vi "Actor Core.vi"(8 "error in":errorcluster, 11 "Chat Window in":refnum<class "Chat Window.lvclass">) -> (0 "error out":errorcluster, 3 "Actor out":refnum<class "Actor.lvclass">)   [LabVIEW 2020, in "Chat Window.lvlib" / "Chat Window.lvclass"]
doc: "(<B>Filename</B>: Actor Framework.lvlib:Actor.lvclass:Actor Core.vi)\n\nReceives messages to the actor, reacts to them, and initiates any error handling that may shut the actor down.\n\nDescendant classes may override this VI to append parallel tasks for the actor to complete while it handles messages. Overrides use the Call Parent Method node."
uses:
  Chat Window.lvclass
  C:/Program Files (x86)/National Instruments/LabVIEW 2020/vi.lib/ActorFramework/Actor/Actor.lvclass
  <vilib>/ActorFramework/Actor/Actor.lvclass
  <vilib>/NI/Actors/Network Endpoint Actors/Notifying Nested Endpoint/Notifying Nested Endpoint.lvclass
  G:/Utilisateurs/hugofroylan.aragon/Documents/Nested Endpoint Actors Optimized/Network Endpoint/Network Endpoint/Network Endpoint.lvclass
  Chat Window.lvclass/Chat Window.ctl
  Nested Endpoint Actors/Network Endpoint/Network Endpoint/Network Endpoint.lvclass/Network Endpoint.ctl
  <vilib>/ActorFramework/Actor/Actor.lvclass/Actor.ctl
  <vilib>/ActorFramework/Message Enqueuer/Message Enqueuer.lvclass/Message Enqueuer.ctl
  Chat Window Messages/Display Text Msg/Display Text Msg.lvclass/Display Text Msg.ctl
  Chat Window Messages/Update Number Msg/Update Number Msg.lvclass/Update Number Msg.ctl
  <vilib>/ActorFramework/Message Enqueuer/Init from Existing Queue.vi
  <vilib>/ActorFramework/Message Enqueuer/Enqueue.vi
  Chat Window Messages/Display Text Msg/Display Text Msg.lvclass
  C:/Program Files (x86)/National Instruments/LabVIEW 2020/vi.lib/ActorFramework/Message/Message.lvclass
  Chat Window Messages/Update Number Msg/Update Number Msg.lvclass
  <vilib>/ActorFramework/Stop Msg/Stop Msg.lvclass
  <vilib>/ActorFramework/Message Priority Queue/Priority Enqueue.vi
  <vilib>/ActorFramework/Message Enqueuer/Message Enqueuer.lvclass
  Nested Endpoint Actors/Network Endpoint/Network Endpoint/Network Endpoint.lvclass
panel:
  out "Text to display 2":string
  in  "Send echo":bool
  out "Number":dbl
  out "Connected":bool
  in  "Send":bool
  out "Text to display":string
  in  "Text to send":string
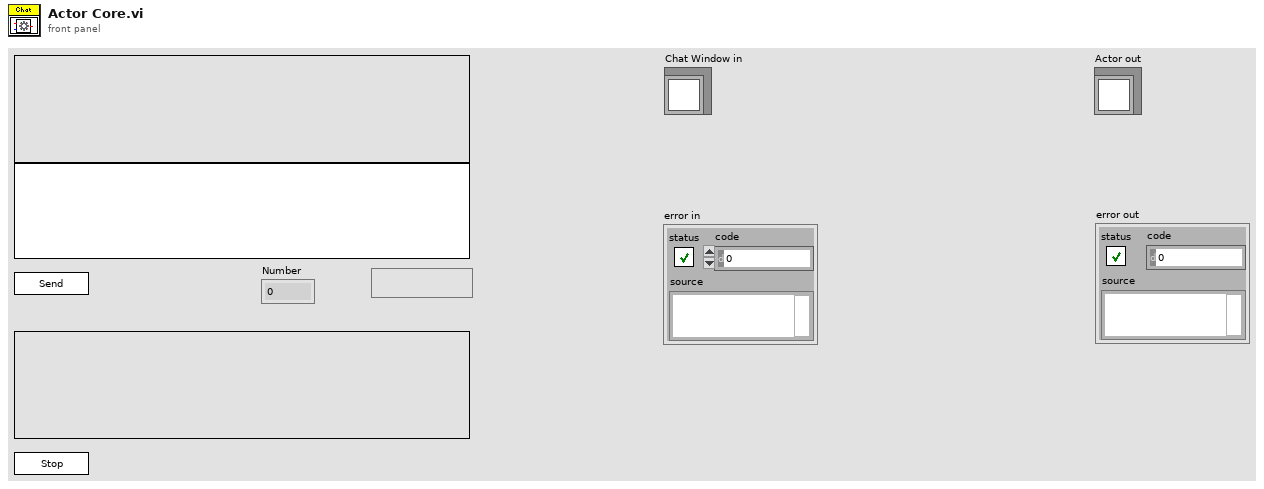
[diagram p1: front panel]
types:
  T1 = cluster{"Stop":refnum<user-event>, "Text":refnum<user-event>, "Connected":refnum<user-event>, "Number":refnum<user-event>, "echo":refnum<user-event>}
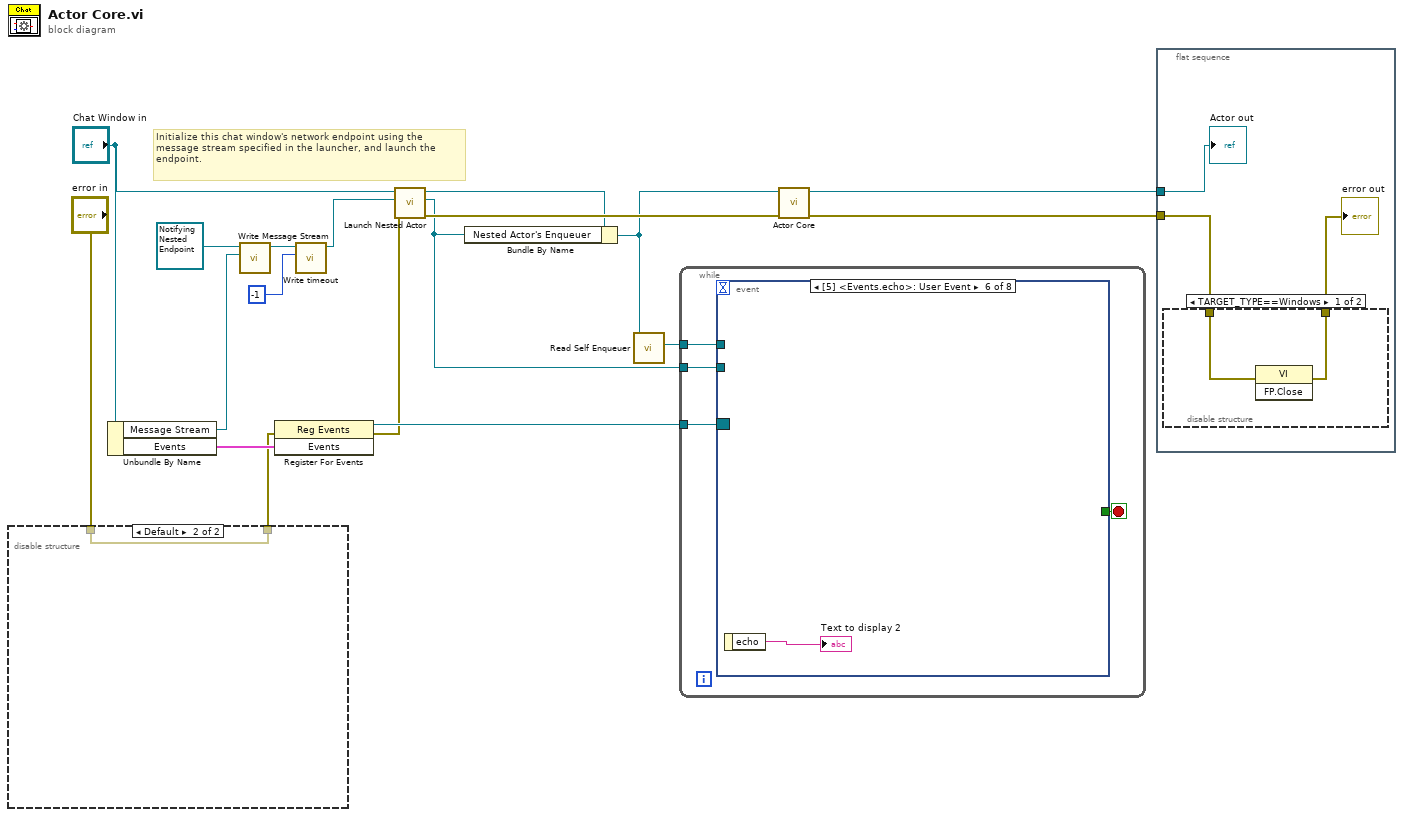
[diagram p0: block diagram]
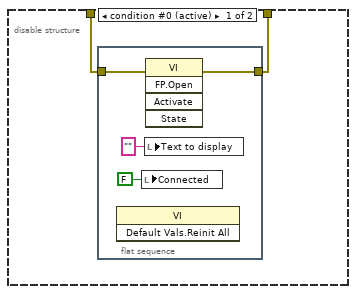
[diagram p2: hidden frame]
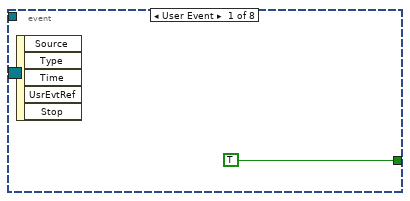
[diagram p4: hidden frame]
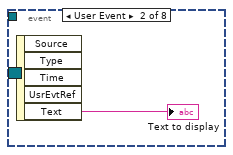
[diagram p5: hidden frame]
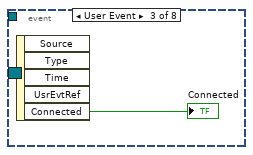
[diagram p6: hidden frame]
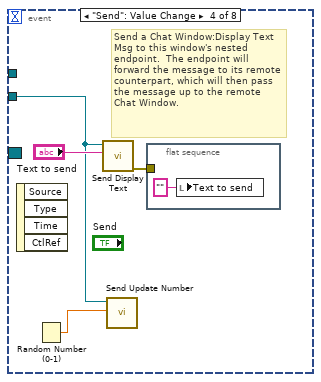
[diagram p7: hidden frame]
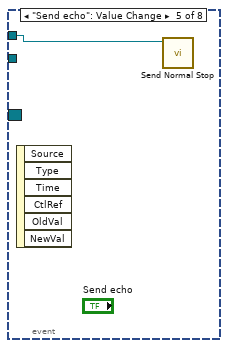
[diagram p8: hidden frame]
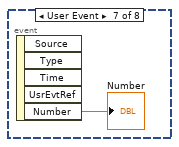
[diagram p9: hidden frame]
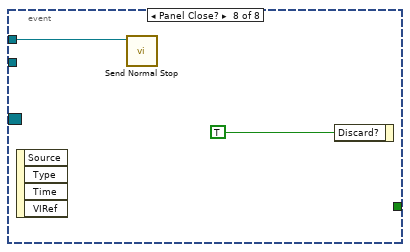
[diagram p10: hidden frame]
diagram:
  # "Initialize this chat window's network endpoint using the message stream specified in the launcher, and launch the endpoint."
  n1 = disable-structure shown="Default" {
    disable-tunnel: [w20 w25] -> w11
    disable-tunnel: "error in" -> [w19 w25]
    frame condition #0 (active) {
      n2 = flat-sequence {
        tunnel: [w24] -> w20
        tunnel: w19 -> [w21]
        frame #0 {
          n3 = invoke class="VI" method="Default Vals.Reinit All"() -> ()  [unwired: 3 in, 3 out]
          n4 = local write "Connected"(FALSE ("Connected")) -> ()
          n5 = local write "Text to display"("" ("Text to display")) -> ()
          n6 = invoke class="VI" method="FP.Open"(error in=w21) -> (error out=w24:errorcluster)  [unwired: 4 in, 4 out]
        }
      }
    }
    frame condition #1 {
    }
  }
  n7 = Unbundle By Name("Chat Window in") -> ("Message Stream"=w12:refnum<class "Message Stream.lvclass">, "Events"=w16:T1)
  n8 = call "Write Message Stream.vi"("Message Stream"=w12, "Network Endpoint in"=refnum<class "Notifying Nested Endpoint.lvclass"> refnum ("Notifying Nested Endpoint.lvclass")) -> ("Network Endpoint out"=w9:refnum<class "Notifying Nested Endpoint.lvclass">)  [unwired: 9 in]
  n9 = register-events(error in=w11, w16) -> (reference out=w15:refnum<event-registration>, error out=w6:errorcluster)  [unwired: 1 in]
  n10 = call "Write timeout.vi"("timeout"=-1, "Network Endpoint in"=w9) -> ("Network Endpoint out"=w4:refnum<class "Notifying Nested Endpoint.lvclass">)  [unwired: 9 in]
  n11 = call <vilib>:"Launch Nested Actor.vi"("error in (no error)"=w6, "Nested Actor"=w4, "Caller Actor in"="Chat Window in") -> ("error out"=w14:errorcluster, "Nested Actor's Enqueuer"=w2:refnum<class "Message Enqueuer.lvclass">, "Caller Actor out"=w3:refnum<class "Chat Window.lvclass">)  [unwired: 6 in]
  n12 = Bundle By Name(cluster=w3, "Nested Actor's Enqueuer"=w2) -> (w1:refnum<class "Chat Window.lvclass">)
  n13 = call <vilib>:"Read Self Enqueuer.vi"("Actor"=w1) -> ("Self Enqueuer"=w10:refnum<class "Message Enqueuer.lvclass">)  [unwired: 10 in]
  n14 = while {
    tunnel: w15 -> [w29]
    tunnel: w2 -> [w27]
    tunnel: w10 -> [w26]
    stop <- w28 stop-if-true
    n15 = event shown="[5] <Events.echo>: User Event" {
      selector: w29 -> [_ _ _ _ _ _ _ _]
      dyn-events: _ -> [_ _ _ _ _ _ _ _]
      timeout: _ -> [_ _ _ _ _ _ _ _]
      tunnel: [TRUE _ _ _ _ _ _ _] -> w28
      tunnel: w27 -> [_ _ _ w34 _ _ _ _]
      tunnel: w26 -> [_ _ _ _ w38 _ _ w41]
      event User Event {
        n16 = event-data() -> ()  [unwired: 1 in, 5 out]
      }
      event User Event {
        n17 = event-data() -> ("Text"=→"Text to display":string)  [unwired: 1 in, 4 out]
      }
      event User Event {
        n18 = event-data() -> ("Connected"=→"Connected":bool)  [unwired: 1 in, 4 out]
      }
      event "Send": Value Change {
        # "Send a Chat Window:Display Text Msg to this window's nested endpoint.  The endpoint will forward the message to its remote counterpart, which will then pass the message up to the remote Chat Window."
        n19 = event-data() -> ()  [unwired: 1 in, 4 out]
        n20 = Random Number (0-1)() -> (number: 0 to 1=w33:dbl)
        n21 = call "Send Display Text.vi"("Text"="Text to send", "Message Enqueuer"=w34) -> ("error out"=w35:errorcluster)  [unwired: 8 in, 1 out]
        n22 = call "Send Update Number.vi"("New number"=w33, "Message Enqueuer"=w34) -> ()  [unwired: 8 in, 2 out]
        n23 = flat-sequence {
          tunnel: w35 -> [_]
          frame #0 {
            n24 = local write "Text to send"("" ("Text to send")) -> ()
          }
        }
      }
      event "Send echo": Value Change {
        n25 = event-data() -> ()  [unwired: 1 in, 6 out]
        n26 = call <vilib>:"Send Normal Stop.vi"("Message Enqueuer"=w38) -> ()  [unwired: 10 in, 1 out]
      }
      event User Event {
        n27 = event-data() -> ("echo"=→"Text to display 2":string)  [unwired: 1 in]
      }
      event User Event {
        n28 = event-data() -> ("Number"=→"Number":dbl)  [unwired: 1 in, 4 out]
      }
      event Panel Close? {
        n29 = event-data() -> ()  [unwired: 1 in, 4 out]
        n30 = call <vilib>:"Send Normal Stop.vi"("Message Enqueuer"=w41) -> ()  [unwired: 10 in, 1 out]
        n31 = event-data("Discard?"=TRUE) -> ()  [unwired: 1 in, 1 out]
      }
    }
  }
  n32 = call-parent "Actor Core.vi"("error in"=w14, "Actor in"=w1) -> ("error out"=w18:errorcluster, "Actor out"=w17:refnum<class "Actor.lvclass">)  [unwired: 8 in]
  n33 = flat-sequence {
    tunnel: w18 -> [w43]
    tunnel: w17 -> [w45]
    frame #0 {
      n34 = disable-structure shown="TARGET_TYPE==Windows" {
        disable-tunnel: w43 -> [w47 _]
        disable-tunnel: [w46 _] -> w44
        frame condition #0 (active) {
          n35 = invoke class="VI" method="FP.Close"(error in=w47) -> (error out=w46:errorcluster)  [unwired: 2 in, 2 out]
        }
        frame condition #1 {
        }
      }
      "error out" <- w44
      "Actor out" <- w45
    }
  }
